vi "Updated Command Status.vi"(8 "error in (no error)":errorcluster, 10 "Command Status":T1, 11 "Command Processor in":refnum<class "Command Processor.lvclass">) -> (0 "error out":errorcluster, 3 "Command Processor out":refnum<class "Command Processor.lvclass">)   [LabVIEW 2013, in "Robot Actors.lvlib" / "Command Processor.lvlib" / "Command Processor.lvclass"]
uses:
  Command Processor.lvclass
  Command/Command Class/Command States.ctl
  Command/Command Class/Command.lvclass
  Command/Command Class/Command Status.ctl
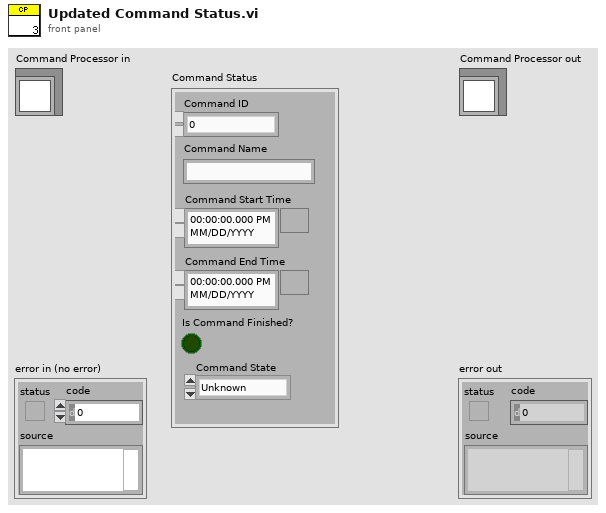
[diagram p1: front panel]
types:
  T1 = typedef "Robot Actors.lvlib/Command.lvlib/Command.lvclass/Command Status.ctl" = cluster{"Command Name":string, "Command Start Time":timestamp, "Command End Time":timestamp, "Is Command Finished?":bool, "Command ID":dbl, "Command State":T2}
  T2 = typedef "Robot Actors.lvlib/Command.lvlib/Command.lvclass/Command States.ctl" = enum16{"Unknown", "Started", "Stopped", "Finished"}
  T3 = typedef "Robot Actors.lvlib/Command Processor.lvlib/Command Processor.lvclass/Command Processor Status.ctl" = cluster{"Next Command ID":dbl, "Current Command Status":T1, "Previous Command Status ":T1}
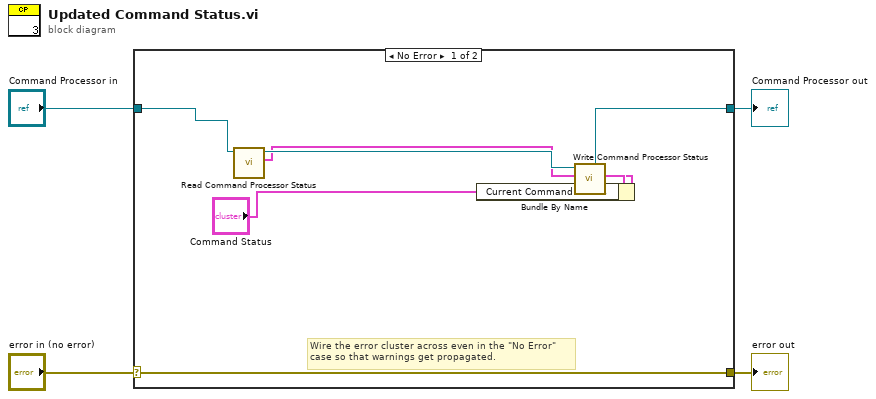
[diagram p0: block diagram]
diagram:
  n1 = case shown="No Error" "error in (no error)" {
    selector: "error in (no error)" -> [w11 w13]
    tunnel: [w11 w13] -> w3
    tunnel: [w9 w12] -> w1
    tunnel: "Command Processor in" -> [w10 w12]
    frame No Error {
      # "Wire the error cluster across even in the \"No Error\"\ncase so that warnings get propagated."
      n2 = call-dynamic "Read Command Processor Status.vi"("Command Processor in"=w10) -> ("Command Processor Status"=w7:T3, "Command Processor out"=w8:refnum<class "Command Processor.lvclass">)  [unwired: 8 in, 1 out]
      n3 = Bundle By Name(cluster=w7, "Current Command Status"="Command Status") -> (w6:T3)
      n4 = call-dynamic "Write Command Processor Status.vi"("Command Processor Status"=w6, "Command Processor in"=w8) -> ("Command Processor out"=w9:refnum<class "Command Processor.lvclass">)  [unwired: 8 in, 1 out]
    }
    frame Error {
    }
  }
  "error out" <- w3
  "Command Processor out" <- w1
